vi "Add Major Frame.vi"(6 "loopCountSpecified (F)":bool, 7 "loopCount (0: continous)":i32, 8 "error in":errorcluster, 9 "Minor Frames":refnum<k24>[](array[refnum]), 10 "name":string, 11 "BusController in":refnum<k24>) -> (0 "error out":errorcluster, 3 "BusController out":refnum<k24>)   [LabVIEW 2020, in "Ballard_1553_Hardware_ni.lvlib"]
uses:
  Ballard_1553_Hardware_ni.lvlib
  C:/Users/Administrator/Desktop/GIT/Ballard-MIL-STD-1553-Custom-Device/Source/System Explorer/SubVIs/Parse XML Ballard/1.2/BTIXML_SerDes.dll
  Ballard-MIL-STD-1553-Custom-Device/Source/System Explorer/SubVIs/Parse XML Ballard/1.2/BTIXML_SerDes.dll
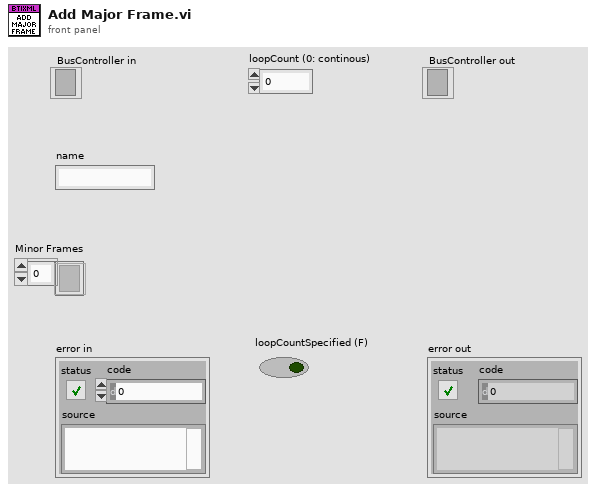
[diagram p1: front panel]
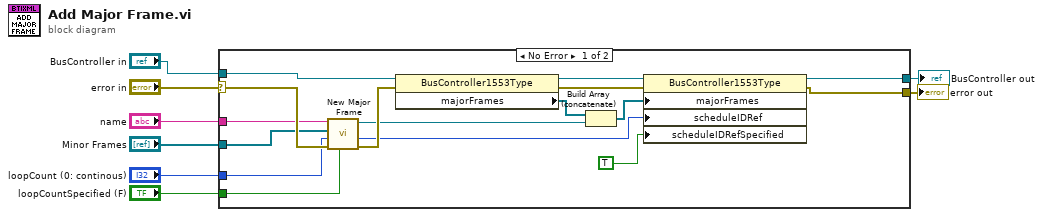
[diagram p0: block diagram]
diagram:
  n1 = case shown="No Error" "error in" {
    selector: "error in" -> [w17 w25]
    tunnel: [w21 w25] -> w8
    tunnel: [w22 w26] -> w7
    tunnel: "BusController in" -> [w24 w26]
    tunnel: "name" -> [w14 _]
    tunnel: "Minor Frames" -> [w13 _]
    tunnel: "loopCount (0: continous)" -> [w12 _]
    tunnel: "loopCountSpecified (F)" -> [w11 _]
    frame No Error {
      n2 = call "New Major Frame.vi"("loopCountSpecified (F)"=w11, "error in"=w17, "loopCount (0: continous)"=w12, "Minor Frames"=w13, "name"=w14) -> ("error out"=w16:errorcluster, "Major Frame ID out"=w10:i32, "new major frame"=w15:refnum<k24>)  [unwired: 4 in]
      n3 = property class="BusController1553Type"(reference=w24, error in=w16) -> (reference out=w23:refnum<k24>, error out=w20:errorcluster, "majorFrames"=w19:refnum<k24>[])
      n4 = Build Array (concatenate)(w19, w15) -> (w18:refnum<k24>[])
      n5 = property class="BusController1553Type"(reference=w23, error in=w20, "majorFrames"=w18, "scheduleIDRef"=w10, "scheduleIDRefSpecified"=TRUE) -> (reference out=w22:refnum<k24>, error out=w21:errorcluster)
    }
    frame Error {
    }
  }
  "error out" <- w8
  "BusController out" <- w7
